vi "Final GRR Calculation.vi"(7 "Test Limits":T2, 8 "Calc Info":T1, 9 "R Double Bar":dbl, 10 "X Bar Diff":dbl, 11 "Rp":dbl) -> (1 "Percent GRR":dbl, 2 "Percent AV":dbl, 3 "Percent EV":dbl)   [LabVIEW 2018, in "GRR Core.lvclass"]
uses:
  GRR Core.lvclass
  TestDataMgr/Typedefs/Test Limits.ctl
  Typedefs/Calculation Info.ctl
  Typedefs/K Coeff.ctl
  TestDataMgr/TestDataMgr.lvclass
panel:
  out "TV":dbl
  out "GRR":dbl
  out "PV":dbl
  out "AV":dbl
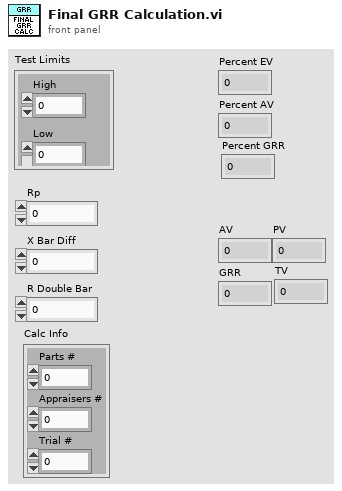
[diagram p1: front panel]
types:
  T1 = typedef "GRR Core.lvclass/Calculation Info.ctl" = cluster{"Parts #":u8, "Appraisers #":u8, "Trial #":u8}
  T2 = typedef "TestDataMgr.lvclass/Test Limits.ctl" = cluster{"High":dbl, "Low":dbl}
  T3 = typedef "GRR Core.lvclass/K Coeff.ctl" = enum16{"K1", "K2 or K3"}
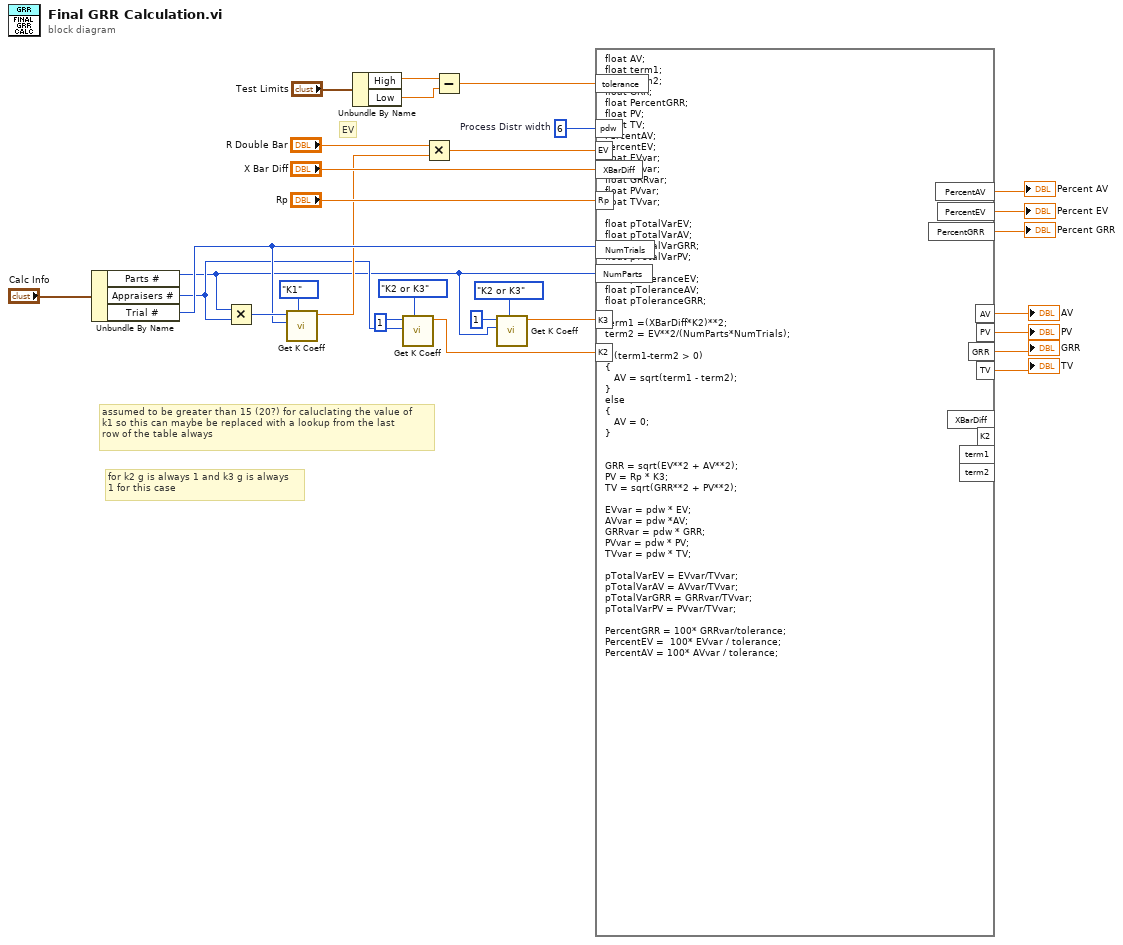
[diagram p0: block diagram]
diagram:
  w21 = 6  # Process Distr width
  # "EV"
  # "for k2 g is always 1 and k3 g is always\n1 for this case"
  # "assumed to be greater than 15 (20?) for caluclating the value of\nk1 so this can maybe be replaced with a lookup from the last\nrow of the table always"
  n1 = Unbundle By Name("Calc Info") -> ("Parts #"=w8:u8, "Appraisers #"=w10:u8, "Trial #"=w13:u8)
  n2 = Multiply(x=w8, y=w10) -> (x*y=w14:u8)
  n3 = call "Get K Coeff.vi"("K Coeff"=K_Coeff."K1", "Number of Trials/Parts"=w13, "G"=w14) -> ("K Coeff"=w12:dbl)  [unwired: 8 in]
  n4 = Unbundle By Name("Test Limits") -> ("High"=w19:dbl, "Low"=w18:dbl)
  n5 = call "Get K Coeff.vi"("K Coeff"=K_Coeff."K2 or K3", "Number of Trials/Parts"=w10, "G"=1 ("Number of Trials")) -> ("K Coeff"=w7:dbl)  [unwired: 8 in]
  n6 = Multiply(x="R Double Bar", y=w12) -> (x*y=w27:dbl)
  n7 = Subtract(x=w19, y=w18) -> (x-y=w17:dbl)
  n8 = call "Get K Coeff.vi"("K Coeff"=K_Coeff."K2 or K3", "Number of Trials/Parts"=w8, "G"=1 ("Number of Trials")) -> ("K Coeff"=w6:dbl)  [unwired: 8 in]
  n9 = formula code="float AV;\nfloat term1;\nfloat term2;\nfloat GRR;\nfloat PercentGRR;\nfloat PV;\nfloat TV;\nPercentAV;\nPercentEV;\nfloat EVvar;\nfloat AVvar;\nfloat GRRvar;\nfloat PVvar;\nfloat TVvar;\n\nfloat pTotalVarEV;\nfloat pTotalVarAV;\nfloat pTotalVarGRR;\nfloat pTotalVarPV;\n\nfloat pToleranceEV;\nfloat pToleranceAV;\nfloat pToleranceGRR;\n\nterm1 =(XBarDiff*K2)**2;\nterm2 = EV**2/(NumParts*NumTrials);\n\nif (term1-term2 > 0)\n{\n   AV = sqrt(term1 - term2);\n}\nelse\n{\n   AV = 0;\n}\n\n\nGRR = sqrt(EV**2 + AV**2);\nPV = Rp * K3;\nTV = sqrt(GRR**2 + PV**2);\n\nEVvar = pdw * EV;\nAVvar = pdw *AV;\nGRRvar = pdw * GRR;\nPVvar = pdw * PV;\nTVvar = pdw * TV;\n\npTotalVarEV = EVvar/TVvar;\npTotalVarAV = AVvar/TVvar;\npTotalVarGRR = GRRvar/TVvar;\npTotalVarPV = PVvar/TVvar;\n\nPercentGRR = 100* GRRvar/tolerance;\nPercentEV =  100* EVvar / tolerance;\nPercentAV = 100* AVvar / tolerance;"("XBarDiff"="X Bar Diff", "K2"=w7, "EV"=w27, "NumParts"=w8, "NumTrials"=w13, "Rp"="Rp", "K3"=w6, "pdw"=w21, "tolerance"=w17) -> ("PercentAV"=→"Percent AV":dbl, "PercentEV"=→"Percent EV":dbl, "PercentGRR"=→"Percent GRR":dbl, "AV"=→"AV":dbl, "PV"=→"PV":dbl, "GRR"=→"GRR":dbl, "TV"=→"TV":dbl)  [unwired: 4 out]
